vi "Read Config.vi"(8 "error in (no error)":errorcluster, 9 "Re-Init?":bool, 10 "ICM File In":path, 11 "No Query in":refnum<class "No Query.lvclass">) -> (0 "error out":errorcluster, 3 "No Query out":refnum<class "No Query.lvclass">)   [LabVIEW 2018, in "No Query.lvclass"]
doc: "No Query.lvclass:Read Config.vi\n\nThis VI reads the No Query Class parameters from the ICM configuration file.\n\nInstrument Communication Module Version 1.0\nDecember, 2017 Original Code Consulting David Thomson\n www.originalcode.com"
uses:
  No Query.lvclass
  No Query.lvclass/No Query.ctl
  Query/Query.lvclass
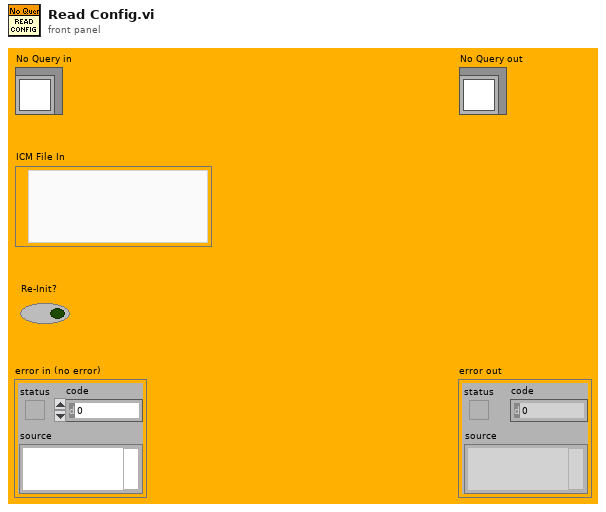
[diagram p1: front panel]
types:
  T1 = typedef "No Query.lvclass/No Queries Config.ctl" = cluster{"null":u32}
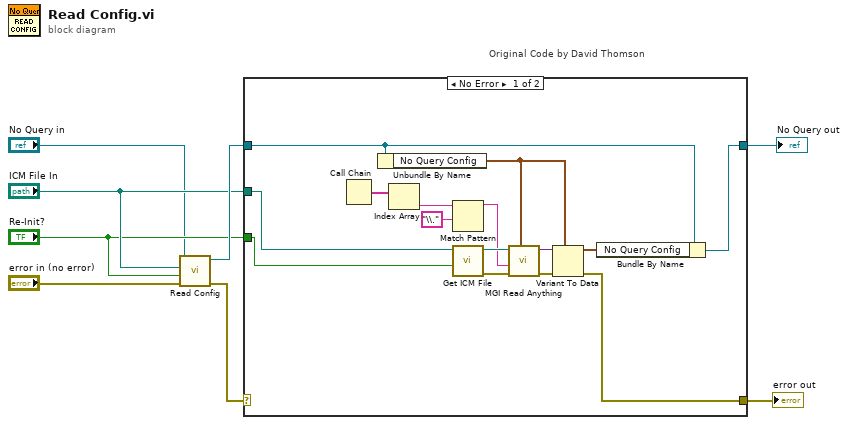
[diagram p0: block diagram]
diagram:
  n1 = call-parent "Read Config.vi"("error in (no error)"="error in (no error)", "Re-Init?"="Re-Init?", "ICM File In"="ICM File In", "Query in"="No Query in") -> ("error out"=w6:errorcluster, "Query out"=w7:refnum<class "No Query.lvclass">)  [unwired: 6 in]
  n2 = case "Original Code by David Thomson" shown="No Error" w6 {
    selector: w6 -> [_ w25]
    tunnel: [w15 w25] -> w4
    tunnel: [w12 w24] -> w5
    tunnel: w7 -> [w11 w24]
    tunnel: "ICM File In" -> [w10 _]
    tunnel: "Re-Init?" -> [w9 _]
    frame No Error {
      n3 = Call Chain() -> (call chain=w20:string[])
      n4 = Unbundle By Name(w11) -> ("No Query Config"=w13:T1)
      n5 = Index Array(array=w20) -> (element=w21:string)  [unwired: 1 in]
      n6 = Match Pattern(string=w21, regular expression="\\.") -> (before substring=w18:string)  [unwired: 1 in, 3 out]
      n7 = call "Get ICM File.vi"("Re-Init?"=w9, "ICM File In"=w10) -> ("error out"=w22:errorcluster, "ICM File"=w23:path)  [unwired: 8 in]
      n8 = call "MGI Read Anything.vi"("Type of Anything"=w13, "Error In"=w22, "Section Name (Name of \"Type of Anything\")"=w18, "Path (dialog)"=w23) -> ("Error Out"=w16:errorcluster, "Anything"=w17:variant)  [unwired: 4 in, 2 out]
      n9 = Variant To Data(error in=w16, type=w13, Variant=w17) -> (data=w14:T1, error out=w15:errorcluster)
      n10 = Bundle By Name(cluster=w11, "No Query Config"=w14) -> (w12:refnum<class "No Query.lvclass">)
    }
    frame Error {
    }
  }
  "error out" <- w4
  "No Query out" <- w5
